vi "testAppBuilder_rt__OutOfBounds.vi"(10 "input":bool) -> ()   [LabVIEW 2014]
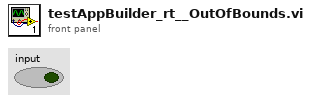
[diagram p1: front panel]
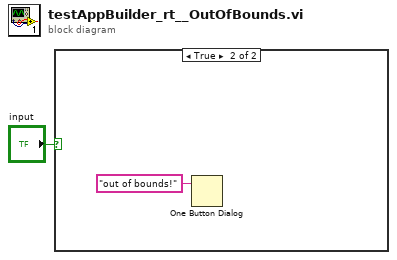
[diagram p0: block diagram]
diagram:
  n1 = case shown="True" "input" {
    frame False {
    }
    frame True {
      n2 = One Button Dialog(message="out of bounds!") -> ()  [unwired: 1 in, 1 out]
    }
  }
